vi "GetAlarms.vi"(0 "DA in":refnum<class "DA.lvclass">, 11 "error in (no error)":errorcluster) -> (4 "DA out":refnum<class "DA.lvclass">, 6 "Alarm":bool, 8 "Warning":bool, 15 "error out":errorcluster)   [LabVIEW 2019, in "DA.lvclass"]
uses:
  DA.lvclass
  DA.lvclass/DA.ctl
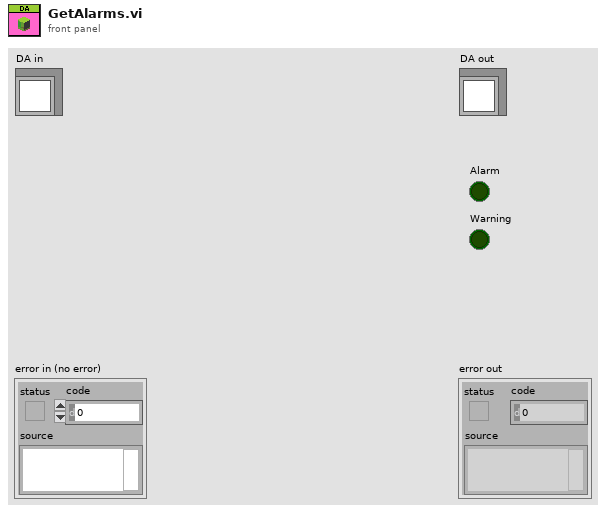
[diagram p1: front panel]
types:
  T1 = typedef "AlarmType.ctl" = enum16{"Normal", "Warning", "Alarm"}
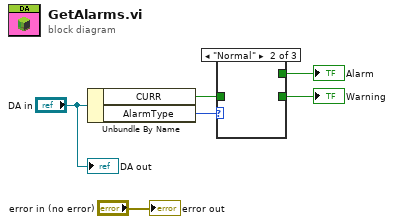
[diagram p0: block diagram]
diagram:
  n1 = Unbundle By Name("DA in") -> ("CURR"=w2:bool, "AlarmType"=w4:T1)
  n2 = case shown="\"Normal\"" w4 {
    tunnel: [w7 _ _] -> w3
    tunnel: w2 -> [w7 _ w8]
    tunnel: [_ _ w8] -> w1
    frame "Alarm" {
    }
    frame "Normal" {
    }
    frame "Warning" {
    }
  }
  "Alarm" <- w3
  "Warning" <- w1
  "error out" <- "error in (no error)"
  "DA out" <- "DA in"
